vi "NI VeriStand - Get Item Path.vi"(8 "error in (no error)":errorcluster, 11 "Item Ref in":T1 format="%.0x") -> (0 "error out":errorcluster, 2 "Path":string, 3 "Item Ref out":T1 format="%.0x", 4 "Found":bool)   [LabVIEW 2020, in "Custom Device Offline API.lvlib"]
uses:
  <vilib>/NI VeriStand/Custom Device Offline API/Custom Device Offline API.lvlib
  <vilib>/NI VeriStand/Custom Device API/Custom Device Item Ref.ctl
  NationalInstruments.VeriStand.SystemDefinitionAPI
  <vilib>/NI VeriStand/Custom Device API/Custom Device API.lvlib
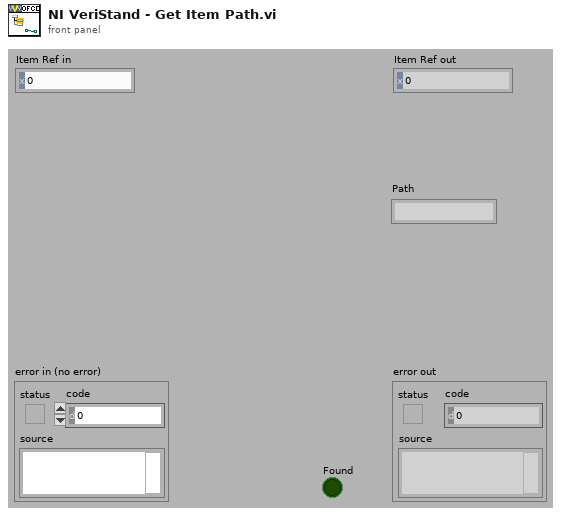
[diagram p1: front panel]
types:
  T1 = typedef "Custom Device API.lvlib/Custom Device Item Ref.ctl" = u64
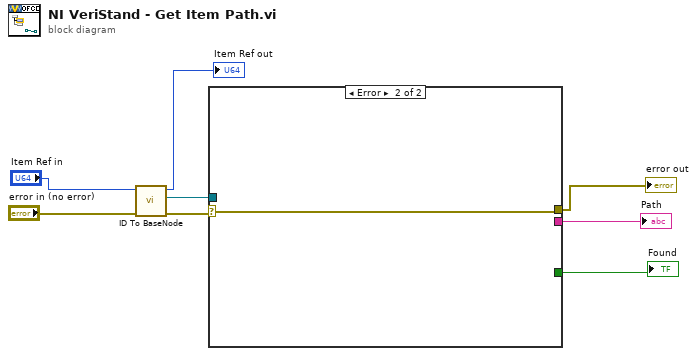
[diagram p0: block diagram]
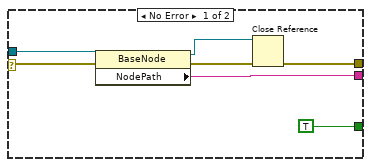
[diagram p2: hidden frame]
diagram:
  n1 = call <vilib>:"ID To BaseNode.vi"("error in (no error)"="error in (no error)", "ID in"="Item Ref in") -> ("error out"=w6:errorcluster, "BaseNode"=w5:refnum<k24>, "ID out"=→"Item Ref out":u64)  [unwired: 7 in]
  n2 = case shown="Error" w6 {
    selector: w6 -> [w14 w16]
    tunnel: w5 -> [w15 _]
    tunnel: [w13 _] -> w4
    tunnel: [w11 w16] -> w3
    tunnel: [TRUE _] -> w2
    frame No Error {
      n3 = property class="BaseNode"(reference=w15, error in=w14) -> (reference out=w10:refnum<k24>, error out=w12:errorcluster, "NodePath"=w13:string)
      n4 = Close Reference(reference=w10, error in (no error)=w12) -> (error out=w11:errorcluster)
    }
    frame Error {
    }
  }
  "error out" <- w3
  "Found" <- w2
  "Path" <- w4
